vi "Convert Filter to Display String.vi"(11 "Filter Info":T1={"Filter Column"=enum."Description", "Filter Type"=enum."Contains", "Filter Value"="", "New Data?"=FALSE, "Enabled?"=FALSE}) -> (3 "String":string)   [LabVIEW 2023, in "VI Properties Editor.lvlib"]
uses:
  VI Properties Editor.lvlib
  CTLs/Filter Info.ctl
  CTLs/Column Name.ctl
  CTLs/Filter Type.ctl
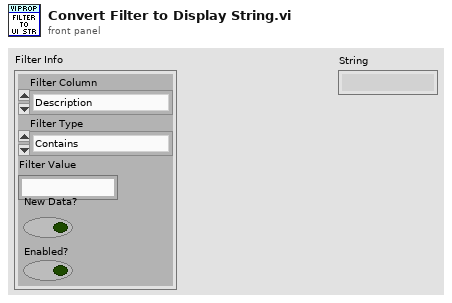
[diagram p1: front panel]
types:
  T1 = typedef "VI Properties Editor.lvlib/Filter Info.ctl" = cluster{"Filter Column":T2, "Filter Type":T3, "Filter Value":string, "New Data?":bool, "Enabled?":bool}
  T2 = typedef "VI Properties Editor.lvlib/Column Name.ctl" = enum16{"Name", "Path", "Type", "Window Title", "Description", "Help Path", "Help Tag", "Custom Title?", "Reentrant?", "Inlined?"}
  T3 = typedef "VI Properties Editor.lvlib/Filter Type.ctl" = enum16{"Contains", "Equals", "Starts with", "Ends with", "Does not contain", "Does not equal", "Is empty", "Is not empty"}
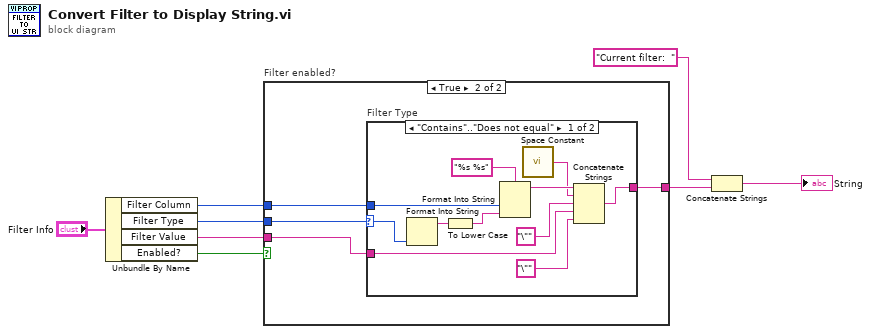
[diagram p0: block diagram]
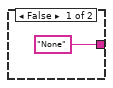
[diagram p2: hidden frame]
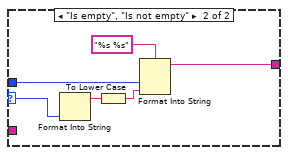
[diagram p3: hidden frame]
diagram:
  n1 = Unbundle By Name("Filter Info") -> ("Filter Column"=w5:T2, "Filter Type"=w7:T3, "Filter Value"=w6:string, "Enabled?"=w4:bool)
  n2 = case "Filter enabled?" shown="True" w4 {
    tunnel: w7 -> [_ w13]
    tunnel: w6 -> [_ w12]
    tunnel: w5 -> [_ w11]
    tunnel: ["None" w10] -> w3
    frame False {
    }
    frame True {
      n3 = case "Filter Type" shown="\"Contains\"..\"Does not equal\"" w13 {
        selector: w13 -> [w21 w27]
        tunnel: w12 -> [w17 _]
        tunnel: w11 -> [w23 w29]
        tunnel: [w14 w28] -> w10
        frame "Contains".."Does not equal" {
          n4 = Format Into String(w21) -> (resulting string=w22:string)  [unwired: 3 in, 1 out]
          n5 = To Lower Case(string=w22) -> (all lower case string=w20:string)
          n6 = Format Into String(format string="%s %s", w23, w20) -> (resulting string=w19:string)  [unwired: 2 in, 1 out]
          n7 = call <vilib>:"Space Constant.vi"() -> ("String"=w18:string)
          n8 = Concatenate Strings(w19, w18, "\"", w17, "\"") -> (w14:string)
        }
        frame "Is empty", "Is not empty" {
          n9 = Format Into String(w27) -> (resulting string=w26:string)  [unwired: 3 in, 1 out]
          n10 = To Lower Case(string=w26) -> (all lower case string=w25:string)
          n11 = Format Into String(format string="%s %s", w29, w25) -> (resulting string=w28:string)  [unwired: 2 in, 1 out]
        }
      }
    }
  }
  n12 = Concatenate Strings("Current filter:  " ("string"), w3) -> (→"String":string)
